vi "Add Context Menu Entry for LV Version.vi"(0 "LabVIEW Version String":string, 5 "LabVIEW EXE Path":path, 11 "error in (no error)":errorcluster) -> (15 "error out":errorcluster)   [LabVIEW 2016]
uses:
  <vilib>/registry/registry.llb/Registry RtKey.ctl
  <vilib>/registry/registry.llb/Write Registry Value Simple STR.vi
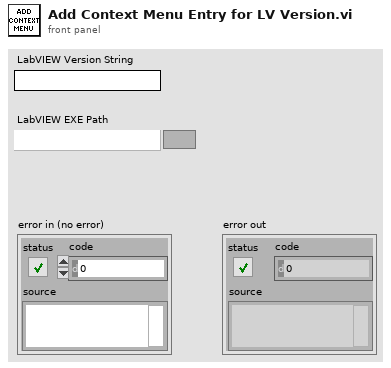
[diagram p1: front panel]
types:
  T1 = typedef "Registry RtKey.ctl" = enum32{"HKEY_CLASSES_ROOT", "HKEY_CURRENT_USER", "HKEY_LOCAL_MACHINE", "HKEY_USERS", "HKEY_PERFORMANCE_DATA", "HKEY_CURRENT_CONFIG", "HKEY_DYN_DATA"}
  T2 = typedef "Registry refnum.ctl" = refnum<k1>
  T3 = cluster{"numSubKeys":i32, "maxSubKeyLen":i32, "maxSubKeyClassLen":i32}
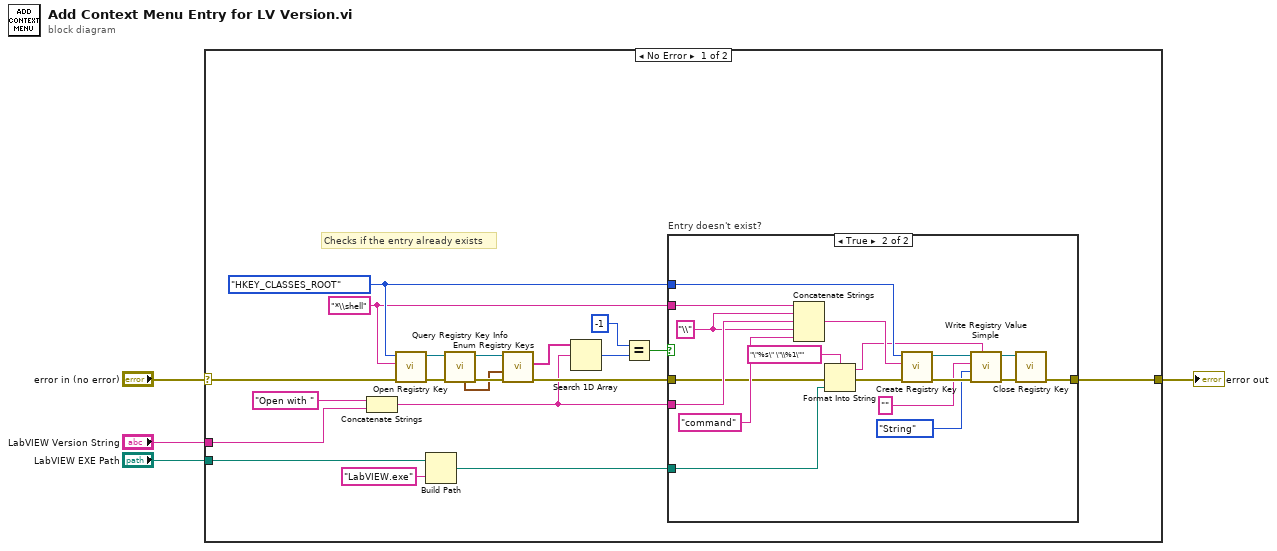
[diagram p0: block diagram]
diagram:
  n1 = case shown="No Error" "error in (no error)" {
    selector: "error in (no error)" -> [w24 w44]
    tunnel: [w23 w44] -> w3
    tunnel: "LabVIEW Version String" -> [w15 _]
    tunnel: "LabVIEW EXE Path" -> [w7 _]
    frame No Error {
      w9 = "*\\shell" ("subkey")
      w10 = Registry_RtKey."HKEY_CLASSES_ROOT" ("root key (HKEY_LOCAL_MACHINE)")
      # "Checks if the entry already exists"
      n2 = Concatenate Strings("Open with ", w15) -> (w8:string)
      n3 = call <vilib>:"Open Registry Key.vi"("error in (no error)"=w24, "subkey"=w9, "root key (HKEY_LOCAL_MACHINE)"=w10) -> ("error out"=w22:errorcluster, "refnum out"=w21:T2)  [unwired: 7 in]
      n4 = Build Path(base path=w7, name or relative path="LabVIEW.exe") -> (appended path=w6:path)
      n5 = call <vilib>:"Query Registry Key Info.vi"("error in (no error)"=w22, "refnum"=w21) -> ("error out"=w20:errorcluster, "refnum out"=w17:T2, "subkey info"=w18:T3)  [unwired: 5 in, 2 out]
      n6 = call <vilib>:"Enum Registry Keys.vi"("error in (no error)"=w20, "subkey info"=w18, "refnum"=w17) -> ("error out"=w19:errorcluster, "subkeys"=w14:string[])  [unwired: 6 in, 1 out]
      n7 = Search 1D Array(1D array=w14, element=w8) -> (index of element=w13:i32)  [unwired: 1 in]
      n8 = Equal?(x=-1, y=w13) -> (x = y?=w11:bool)
      n9 = case "Entry doesn't exist?" shown="True" w11 {
        tunnel: [w25 w33] -> w23
        tunnel: w19 -> [w25 w31]
        tunnel: w10 -> [_ w43]
        tunnel: w9 -> [_ w42]
        tunnel: w8 -> [_ w41]
        tunnel: w6 -> [_ w28]
        frame False {
        }
        frame True {
          w39 = "\\" ("string")
          n10 = Concatenate Strings(w42, w39, w41, w39, "command" ("string")) -> (w40:string)
          n11 = Format Into String(format string="\"%s\" \"\\%1\"", error in=w31, w28) -> (resulting string=w27:string, error out=w30:errorcluster)  [unwired: 1 in]
          n12 = call <vilib>:"Create Registry Key.vi"("error in (no error)"=w30, "subkey"=w40, "root key (HKEY_LOCAL_MACHINE)"=w43) -> ("error out"=w37:errorcluster, "refnum out"=w36:T2)  [unwired: 6 in, 1 out]
          n13 = call-poly <vilib>:"Write Registry Value Simple.vi"("String/Binary data"=w27, "error in (no error)"=w37, "simple data type"=enum16{"String", "Binary", "DWORD"}."String", "value"="", "refnum"=w36) -> ("error out"=w34:errorcluster, "refnum out"=w32:T2)  [unwired: 3 in]
          n14 = call <vilib>:"Close Registry Key.vi"("error in (no error)"=w34, "refnum"=w32) -> ("error out"=w33:errorcluster)  [unwired: 5 in]
        }
      }
    }
    frame Error {
    }
  }
  "error out" <- w3
